vi "Reinitialize.vi"(8 "error in (no error)":errorcluster, 11 "MODBUS in":refnum<class "PL Modbus Client.lvclass">) -> (0 "error out":errorcluster, 3 "MODBUS out":refnum<class "PL Modbus Client.lvclass">)   [LabVIEW 2015, in "PL Modbus Client.lvclass"]
doc: "Reinitializes connection to Modbus server based on previously specified settings."
uses:
  PL Modbus Client.lvclass
  PL Modbus Client.lvclass/PL Modbus Client.ctl
  <vilib>/Instr/_visa.llb/VISA Configure Serial Port (Instr).vi
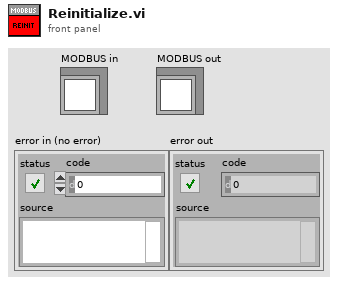
[diagram p1: front panel]
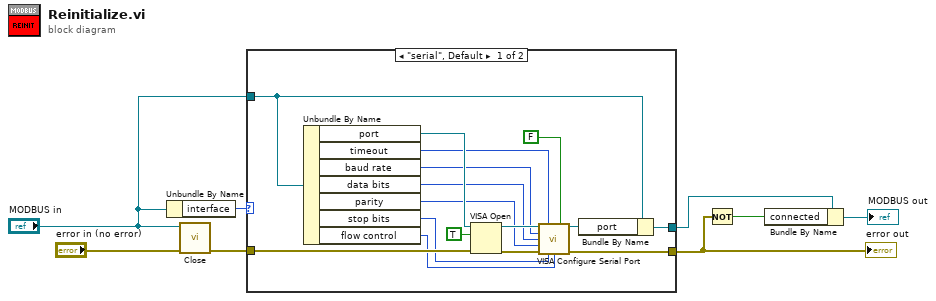
[diagram p0: block diagram]
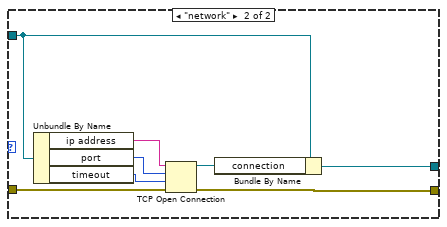
[diagram p2: hidden frame]
diagram:
  n1 = Unbundle By Name("MODBUS in") -> ("interface"=w7:enum16{"serial", "network"})
  n2 = call-dynamic "Close.vi"("error in (no error)"="error in (no error)", "MODBUS in"="MODBUS in") -> ("error out"=w6:errorcluster)  [unwired: 9 in]
  n3 = case shown="\"serial\", Default" w7 {
    tunnel: [w10 w26] -> w1
    tunnel: [w24 w31] -> w5
    tunnel: "MODBUS in" -> [w21 w30]
    tunnel: w6 -> [w22 w29]
    frame "serial", Default {
      n4 = Unbundle By Name(w21) -> ("port"=w20:refnum<visa-resource-name>, "timeout"=w14:u32, "baud rate"=w18:u32, "data bits"=w17:u16, "parity"=w16:u16, "stop bits"=w13:u16, "flow control"=w12:u16)
      n5 = VISA Open(duplicate session (F)=TRUE, error in (no error)=w22, VISA resource name=w20) -> (VISA resource name=w19:refnum<visa-resource-name>, error out=w15:errorcluster)  [unwired: 2 in]
      n6 = call-poly "VISA Configure Serial Port"("VISA resource name"=w19, "timeout (10sec)"=w14, "Enable Termination\nChar (T)"=FALSE ("Enable Termination\nChar (T)"), "baud rate (9600)"=w18, "data bits (8)"=w17, "parity (0:none)"=w16, "error in (no error)"=w15, "stop bits (10: 1 bit)"=w13, "flow control (0:none)"=w12) -> ("VISA resource name out"=w11:refnum<visa-resource-name>, "error out"=w10:errorcluster)  [unwired: 5 in]
      n7 = Bundle By Name(cluster=w21, "port"=w11) -> (w24:refnum<class "PL Modbus Client.lvclass">)
    }
    frame "network" {
      n8 = Unbundle By Name(w30) -> ("ip address"=w25:string, "port"=w27:u16, "timeout"=w28:u32)
      n9 = TCP Open Connection(address=w25, remote port or service name=w27, timeout ms (60000)=w28, error in (no error)=w29) -> (connection ID=w32:refnum<k5>, error out=w26:errorcluster)  [unwired: 1 in]
      n10 = Bundle By Name(cluster=w30, "connection"=w32) -> (w31:refnum<class "PL Modbus Client.lvclass">)
    }
  }
  "error out" <- w1
  n11 = Not(x=w1) -> (.not. x?=w4:bool)
  n12 = Bundle By Name(cluster=w5, "connected"=w4) -> (→"MODBUS out":refnum<class "PL Modbus Client.lvclass">)
